vi "calculatePosVelAccFromLasers.vi"(10 "Right Now":timestamp, 11 "Laser Readings":T2) -> (2 "Positions":dbl[](array[numeric]), 3 "Position Calculations":T1[](array[typedef])=[{"Position (m)"=0.0, "Velocity (m/s)"=0.0, "Acceleration (m/s^2)"=0.0}, {"Position (m)"=0.0, "Velocity (m/s)"=0.0, "Acceleration (m/s^2)"=0.0}, {"Position (m)"=1.276743254418892, "Velocity (m/s)"=0.0, "Acceleration (m/s^2)"=0.0}, {"Position (m)"=1.276743254418892, "Velocity (m/s)"=0.0, "Acceleration (m/s^2)"=0.0}])   [LabVIEW 2017]
uses:
  Type Defs/allLaserReadings.ctl
  Type Defs/laserReading.ctl
  Type Defs/positionData.ctl
panel:
  in  "Distance between Tube Stripes":dbl=30.49
  out "Acceleration (m/s^2)":dbl(graph)
  out "Velocity (m/s)":dbl(graph)
  in  "Stripes per rotation":dbl=1.0
  in  "Wheel Diameter (m)":dbl=0.2032
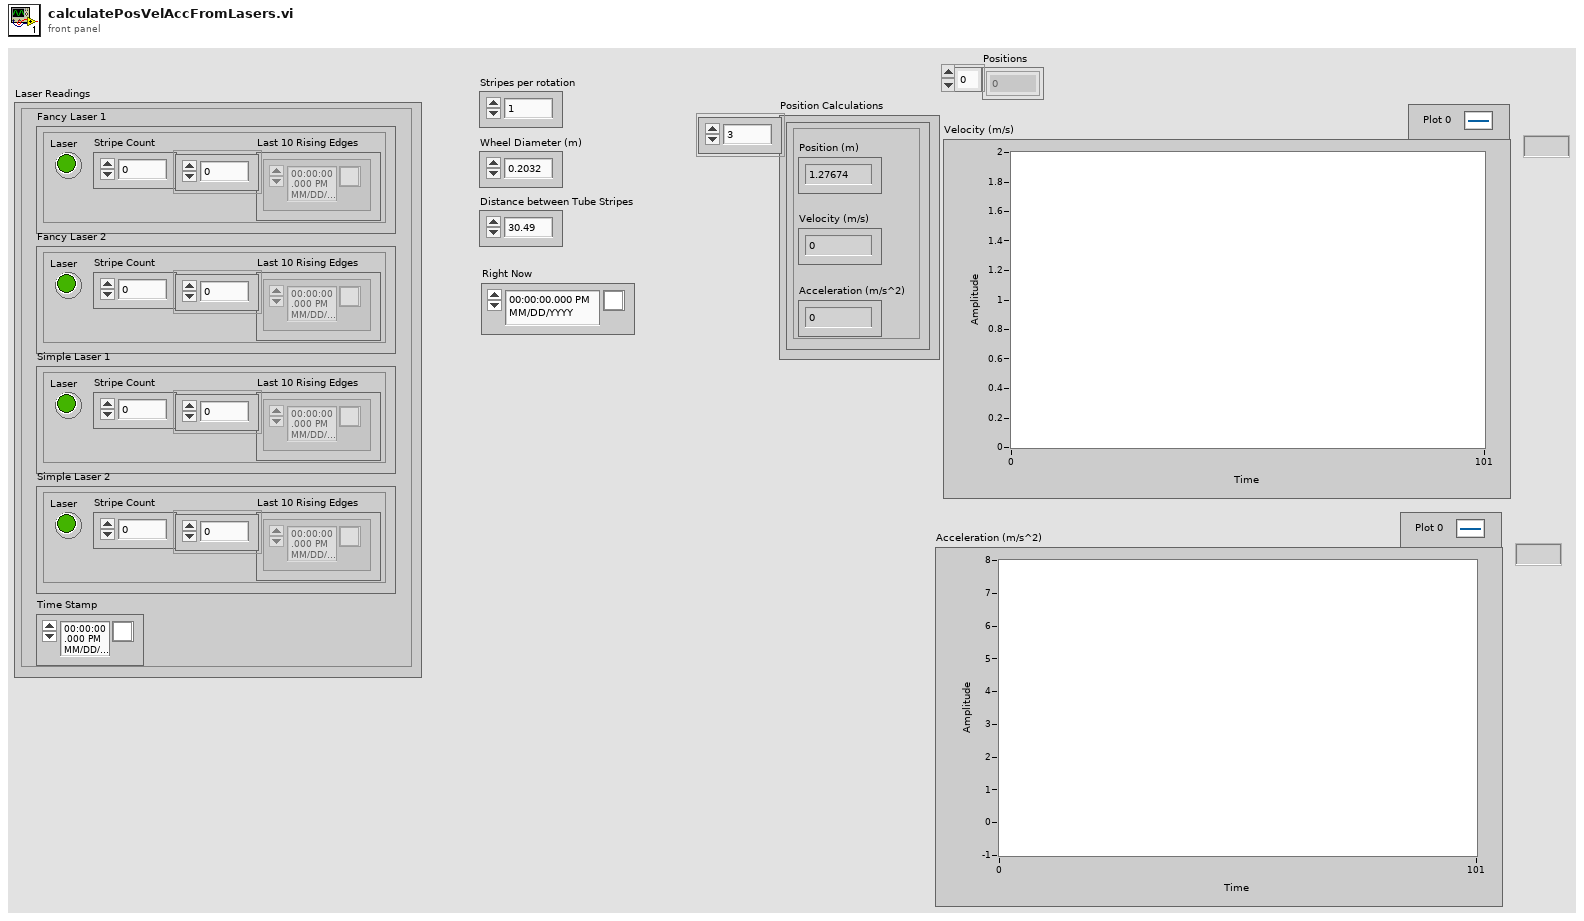
[diagram p1: front panel]
types:
  T1 = typedef "positionData.ctl" = cluster{"Position (m)":dbl, "Velocity (m/s)":dbl, "Acceleration (m/s^2)":dbl}
  T2 = typedef "allLaserReadings.ctl" = cluster{"Fancy Laser 1":T3, "Fancy Laser 2":T3, "Simple Laser 1":T3, "Simple Laser 2":T3, "Time Stamp":timestamp}
  T3 = typedef "laserReading.ctl" = cluster{"Laser":bool, "Stripe Count":u32, "Last 10 Rising Edges":timestamp[]}
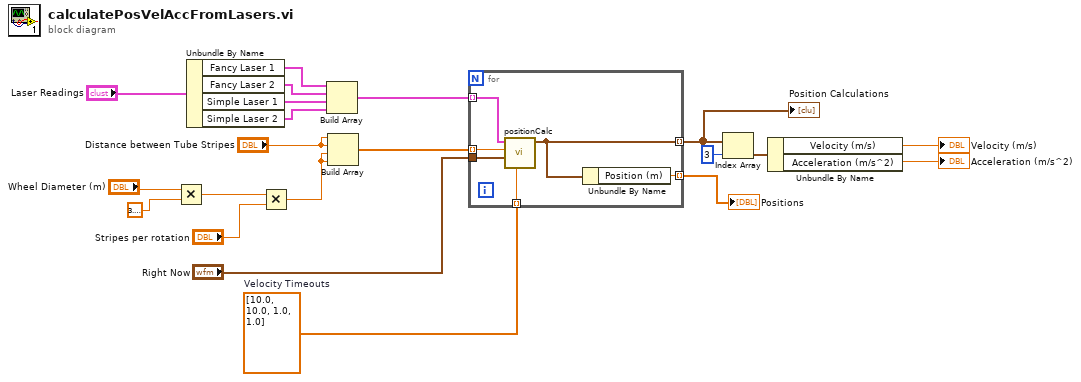
[diagram p0: block diagram]
diagram:
  w2 = dbl[] [10.0, 10.0, 1.0, 1.0]  # Velocity Timeouts
  n1 = Multiply(x="Wheel Diameter (m)", y=3.141592653589793) -> (x*y=w17:dbl)
  n2 = Unbundle By Name("Laser Readings") -> ("Fancy Laser 1"=w16:T3, "Fancy Laser 2"=w15:T3, "Simple Laser 1"=w14:T3, "Simple Laser 2"=w13:T3)
  n3 = Multiply(x=w17, y="Stripes per rotation") -> (x*y=w11:dbl)
  n4 = Build Array(w16, w15, w14, w13) -> (w9:T3[])
  n5 = Build Array("Distance between Tube Stripes", "Distance between Tube Stripes", w11, w11) -> (w10:dbl[])
  n6 = for {
    tunnel: [w23] -> w3 mode=indexing
    tunnel: w10 -> [w27] mode=indexing
    tunnel: w9 -> [w26] mode=indexing
    tunnel: "Right Now" -> [w25]
    tunnel: w2 -> [w24] mode=indexing
    tunnel: [w22] -> w1 mode=indexing
    n7 = call "positionCalc.vi"("Velocity Timeout (s)"=w24, "Right Now"=w25, "Distance per Stripe (m)"=w27, "Laser"=w26) -> ("Position Data"=w23:T1)  [unwired: 7 in]
    n8 = Unbundle By Name(w23) -> ("Position (m)"=w22:dbl)
  }
  "Position Calculations" <- w3
  "Positions" <- w1
  n9 = Index Array(array=w3, index=3) -> (element=w6:T1)
  n10 = Unbundle By Name(w6) -> ("Velocity (m/s)"=→"Velocity (m/s)":dbl, "Acceleration (m/s^2)"=→"Acceleration (m/s^2)":dbl)
